vi "svfa_Apply Overlap.vi"(6 "restart":bool, 8 "error in (no error)":errorcluster, 9 "required block size":i32=-1, 10 "overlap (%)":dbl, 11 "continuous data in":waveform(dbl)) -> (0 "error out":errorcluster, 3 "overlapped blocks out":waveform(dbl)[](array[waveform]))   [LabVIEW 2017]
uses:
  <vilib>/addons/_NISVFA/_Shared subVIs/Common/svc_Check for Waveform Parameter Continuity (no state).vi
  <vilib>/addons/_NISVFA/_Shared subVIs/Common/svc_Get SV Channel Info.vi
  <vilib>/addons/_NISVFA/_Shared subVIs/Common/svc_Engineering Units to Unit Label.vi
  <vilib>/addons/_NISVFA/_Shared subVIs/Common/svc_Unit Label to Engineering Units.vi
panel:
  out "actual block size":i32
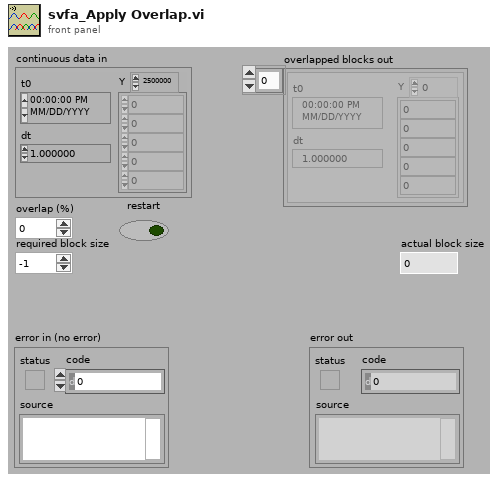
[diagram p1: front panel]
types:
  T1 = cluster{"ignore dt":bool, "ignore t0 continuity":bool, "ignore array length":bool, "ignore channel info":bool, "ignore channel name":bool}
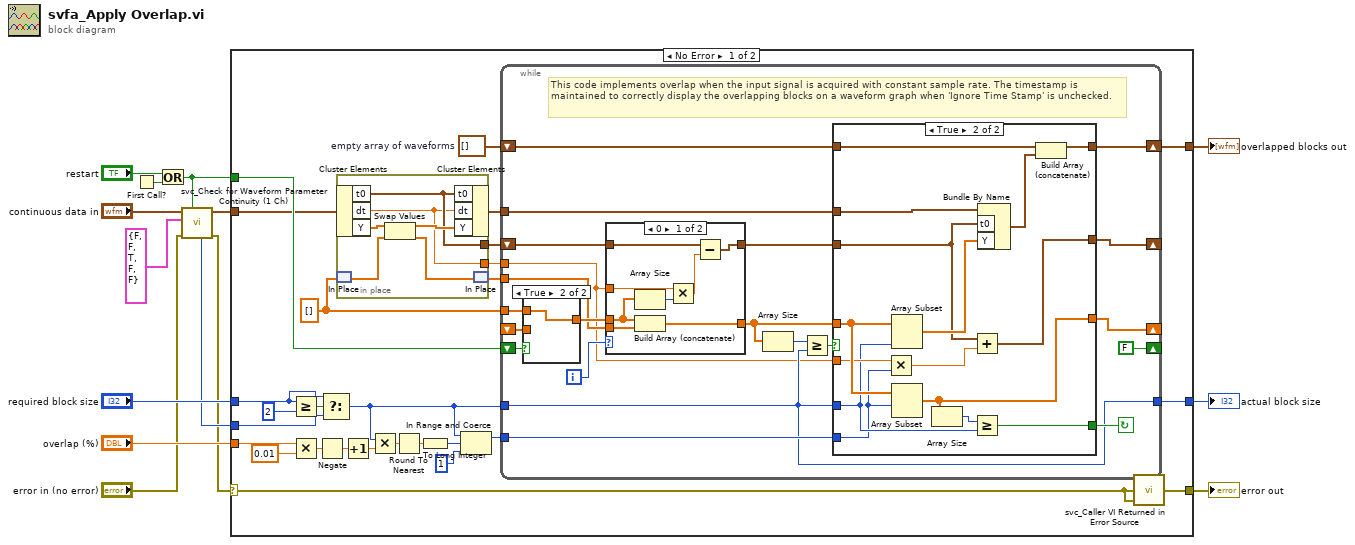
[diagram p0: block diagram]
diagram:
  n1 = First Call?() -> (First Call?: T/F=w13:bool)
  n2 = Or(x="restart", y=w13) -> (x .or. y?=w6:bool)
  n3 = call <vilib>:"svc_Check for Waveform Parameter Continuity (1 Ch).vi"("restart averaging (F)"=w6, "error in (no error)"="error in (no error)", "checks for channel parameter change"=T1 {"ignore dt"=FALSE, "ignore t0 continuity"=FALSE, "ignore array length"=TRUE, "ignore channel info"=FALSE, "ignore channel name"=FALSE} ("parameter controls"), "scaled signal [EU]"="continuous data in") -> ("error out"=w2:errorcluster, "dup scaled signal [EU]"=w4:waveform(dbl), "array length"=w8:i32)  [unwired: 2 in, 3 out]
  n4 = case shown="No Error" w2 {
    selector: w2 -> [w16 w100]
    tunnel: [w40 _] -> w14
    tunnel: "required block size" -> [w31 _]
    tunnel: "overlap (%)" -> [w30 _]
    tunnel: [w28 _] -> w10
    tunnel: w8 -> [w26 _]
    tunnel: w6 -> [w21 _]
    tunnel: w4 -> [w20 _]
    tunnel: [w15 w100] -> w1
    frame No Error {
      w22 = dbl[] [] ("Y")
      w41 = waveform(dbl)[] []  # empty array of waveforms
      n5 = Greater Or Equal?(x=w31, y=2 ("lower limit")) -> (x >= y?=w39:bool)
      n6 = Multiply(x=w30, y=0.01) -> (x*y=w36:dbl)
      n7 = Negate(x=w36) -> (-x=w32:dbl)
      n8 = Select(t=w31, s=w39, f=w26) -> (s? t:f=w17:i32)
      n9 = in-place {
        in-place-border: [w42] -> w27
        in-place-border: [w43] -> w24
        n10 = in-place-cluster #1(w20) -> ("t0"=w43:timestamp, "dt"=w42:dbl, "Y"=w47:dbl[])
        n11 = in-place-match #2(w22) -> (w45:dbl[])
        n12 = Swap Values(12:w47, 14:w45) -> (1:w46:dbl[], 3:w44:dbl[])  [unwired: 1 in]
        n13 = in-place-cluster #1("t0"=w43, "dt"=w42, "Y"=w46) -> (w23:waveform(dbl))
        n14 = in-place-match #2(w44) -> (w25:dbl[])
      }
      n15 = Increment(x=w32) -> (x+1=w33:dbl)
      n16 = Multiply(x=w17, y=w33) -> (x*y=w34:dbl)
      n17 = Round To Nearest(number=w34) -> (nearest integer value=w35:dbl)
      n18 = To Long Integer(number=w35) -> (32bit integer=w29:i32)
      n19 = In Range and Coerce(upper limit=w17, x=w29, lower limit=1) -> (coerced(x)=w19:i32)  [unwired: 1 out]
      n20 = while {
        shift-right: [w67] -> _
        shift-left: _ -> [w68]
        shift-right: [w61] -> _
        shift-left: w24 -> [w51]
        shift-right: [FALSE] -> _
        shift-left: w21 -> [w48]
        shift-right: [w66] -> w40
        shift-left: w41 -> [w64]
        tunnel: w17 -> [w56]
        tunnel: w23 -> [w62]
        tunnel: w25 -> [w53]
        tunnel: w27 -> [w49]
        tunnel: w19 -> [w60]
        tunnel: w22 -> [w59]
        tunnel: [w56] -> w28
        i -> [w55]
        stop <- w63 continue-if-true
        # "This code implements overlap when the input signal is acquired with constant sample rate. The timestamp is maintained to correctly display the overlapping blocks on a waveform graph when 'Ignore Time Stamp' is unchecked."
        n21 = case shown="True" w48 {
          tunnel: w68 -> [w69 _]
          tunnel: w59 -> [_ w70]
          tunnel: [w69 w70] -> w54
          frame False {
          }
          frame True {
          }
        }
        n22 = case shown="0" w55 {
          tunnel: w54 -> [w76 w80]
          tunnel: w53 -> [w78 _]
          tunnel: [w77 w80] -> w52
          tunnel: w49 -> [w75 _]
          tunnel: w51 -> [w73 w79]
          tunnel: [w71 w79] -> w50
          frame 0 {
            n23 = Array Size(array=w76) -> (size(s)=w74:i32)
            n24 = Build Array (concatenate)(w76, w78) -> (w77:dbl[])
            n25 = Multiply(x=w75, y=w74) -> (x*y=w72:dbl)
            n26 = Subtract(x=w73, y=w72) -> (x-y=w71:timestamp)
          }
          frame Default {
          }
        }
        n27 = Array Size(array=w52) -> (size(s)=w58:i32)
        n28 = Greater Or Equal?(x=w58, y=w56) -> (x >= y?=w57:bool)
        n29 = case shown="True" w57 {
          selector: w57 -> [w81 _]
          tunnel: [w82 w85] -> w67
          tunnel: [w83 w99] -> w66
          tunnel: w64 -> [w83 w98]
          tunnel: [w81 w97] -> w63
          tunnel: w52 -> [w82 w94]
          tunnel: w62 -> [_ w91]
          tunnel: [w84 w90] -> w61
          tunnel: w49 -> [_ w89]
          tunnel: w60 -> [_ w86]
          tunnel: w56 -> [_ w87]
          tunnel: w50 -> [w84 w88]
          frame False {
          }
          frame True {
            n30 = Multiply(x=w89, y=w86) -> (x*y=w92:dbl)
            n31 = Array Subset(array=w94, length=w87) -> (w95:dbl[])  [unwired: 1 in]
            n32 = Array Subset(array=w94, index=w86) -> (w85:dbl[])  [unwired: 1 in]
            n33 = Array Size(array=w85) -> (size(s)=w93:i32)
            n34 = Add(x=w88, y=w92) -> (x+y=w90:timestamp)
            n35 = Greater Or Equal?(x=w93, y=w87) -> (x >= y?=w97:bool)
            n36 = Bundle By Name(cluster=w91, "t0"=w88, "Y"=w95) -> (w96:waveform(dbl))
            n37 = Build Array (concatenate)(w98, w96) -> (w99:waveform(dbl)[])
          }
        }
      }
      n38 = call <vilib>:"svc_Caller VI Returned in Error Source.vi"("warning input to caller"=w16, "error in (no error)"=w16) -> ("error out"=w15:errorcluster)  [unwired: 3 in]
    }
    frame Error {
    }
  }
  "overlapped blocks out" <- w14
  "actual block size" <- w10
  "error out" <- w1
